vi "Write SSL Protocols.vi"(8 "error in (no error)":errorcluster, 10 "SSL Protocols":i32[](array[ring])=[240] items=["None"=0, "Ssl2"=12, "Ssl3"=48, "Tls"=192, "Default"=240, "Tls11"=768, "Tls12"=3072], 11 "dotNET SSL Socket in":refnum<class "dotNET SSL Socket.lvclass">) -> (0 "error out":errorcluster, 3 "dotNET SSL Socket out":refnum<class "dotNET SSL Socket.lvclass">)   [LabVIEW 2013, in "dotNET SSL Socket.lvlib" / "dotNET SSL Socket.lvclass"]
uses:
  dotNET SSL Socket.lvclass
  dotNET SSL Socket.lvclass/dotNET SSL Socket.ctl
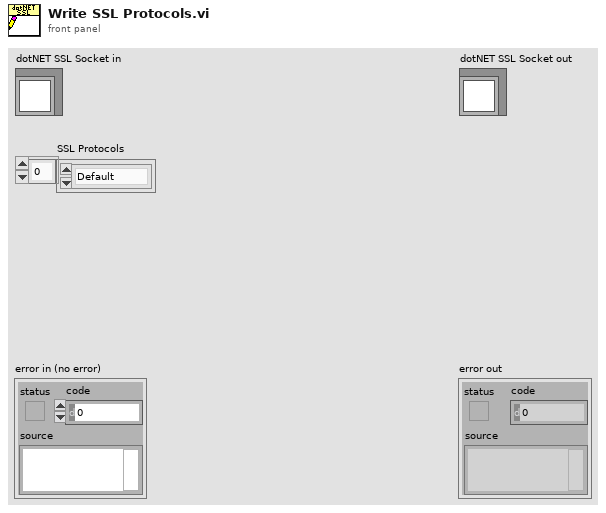
[diagram p1: front panel]
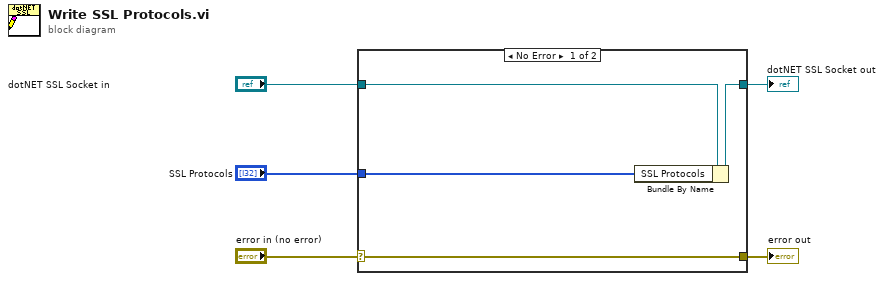
[diagram p0: block diagram]
diagram:
  n1 = case shown="No Error" "error in (no error)" {
    selector: "error in (no error)" -> [w9 w10]
    tunnel: [w9 w10] -> w4
    tunnel: [w7 w11] -> w2
    tunnel: "dotNET SSL Socket in" -> [w8 w11]
    tunnel: "SSL Protocols" -> [w6 _]
    frame No Error {
      n2 = Bundle By Name(cluster=w8, "SSL Protocols"=w6) -> (w7:refnum<class "dotNET SSL Socket.lvclass">)
    }
    frame Error {
    }
  }
  "error out" <- w4
  "dotNET SSL Socket out" <- w2
